vi "Persistent_New_6x8x6.vi"(0 "reference in":refnum<class "G4BaseTemplate_Simple_4x4x4.lvclass">, 1 "Object name":string, 5 "error in (no error)":errorcluster, 6 "CreateMethod(Create or look up existing)":T1(ring), 7 "Persistent/Debugging(Default)":enum16{"Default", "Persistent", "NonPersistent"}(ring)) -> (14 "reference out":refnum<class "G4BaseTemplate_Simple_4x4x4.lvclass">, 15 "NewObjectCreated":bool, 16 "DVRRefOut":refnum<data-value>, 19 "error out":errorcluster)   [LabVIEW 2014]
doc: "..\\..\\..\\..\\Provider_EndevoGOOP400\\Templates\\G4BaseTemplate_Simple_4x4x4\\G4BaseTemplate_Simple_4x4x4.lvclass"
uses:
  <resource>/Framework/Providers/Open_GDS/ClassProviders/Provider_EndevoGOOP400/Templates/G4BaseTemplate_Simple_4x4x4/G4BaseTemplate_Simple_4x4x4.lvclass
  <resource>/Framework/Providers/Open_GDS/ClassProviders/Provider_EndevoGOOP400/Templates/G4BaseTemplate_Simple_4x4x4/protected/ObjectAttributes.ctl
panel:
  in  "DVRRef(Hidden)":refnum<data-value>
  in  "Data":T2 {"Attribute1" format="%.2f"}
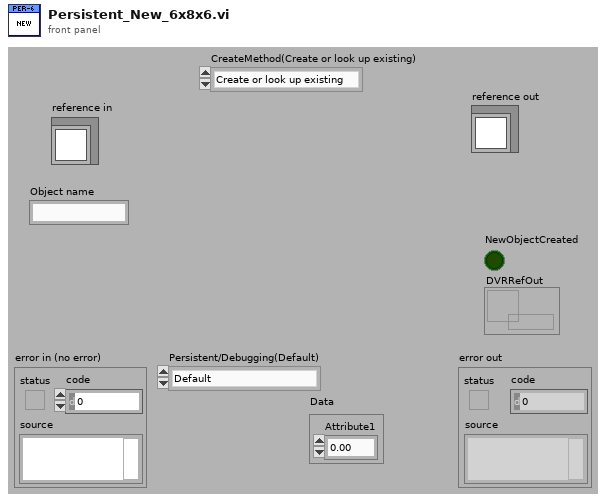
[diagram p1: front panel]
types:
  T1 = enum16{"Create or look up existing", "Look up existing"}
  T2 = typedef "G4BaseTemplate_Simple_4x4x4.lvclass/ObjectAttributes.ctl" = cluster{"Attribute1":dbl}
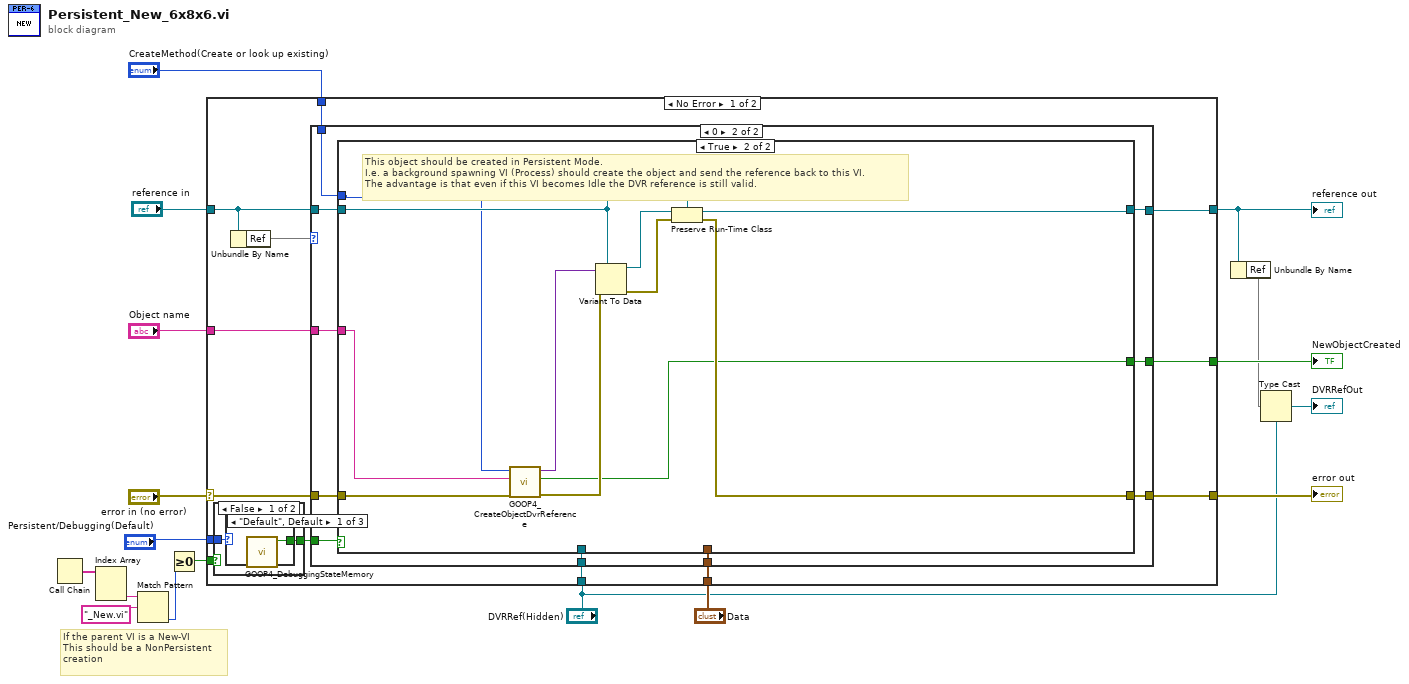
[diagram p0: block diagram]
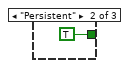
[diagram p2: hidden frame]
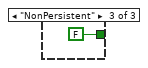
[diagram p3: hidden frame]
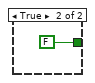
[diagram p4: hidden frame]
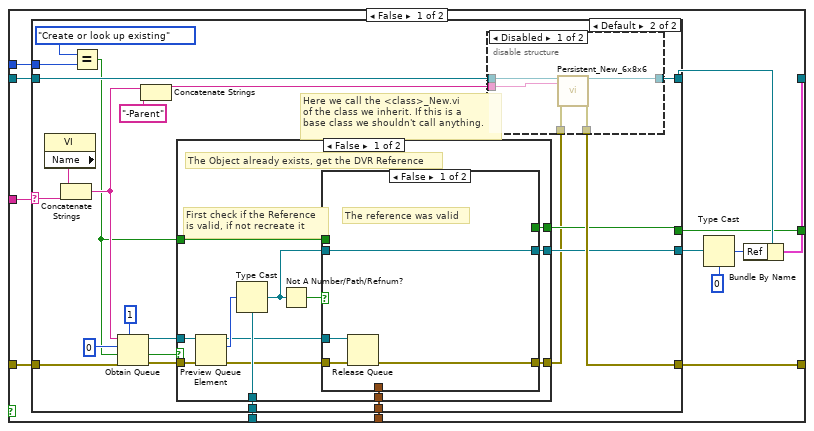
[diagram p6: hidden frame]
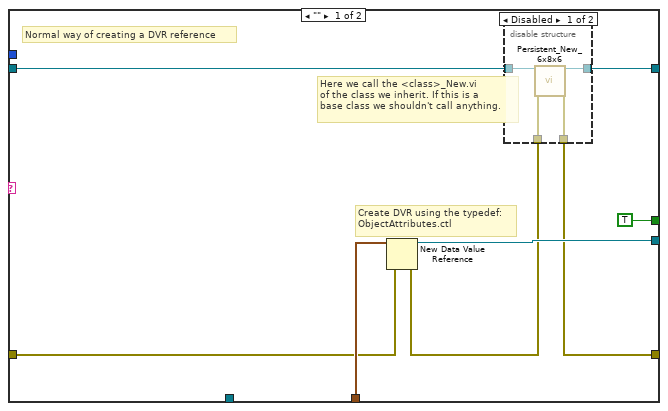
[diagram p7: hidden frame]
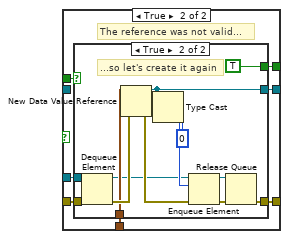
[diagram p9: hidden frame]
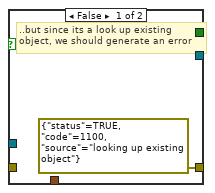
[diagram p10: hidden frame]
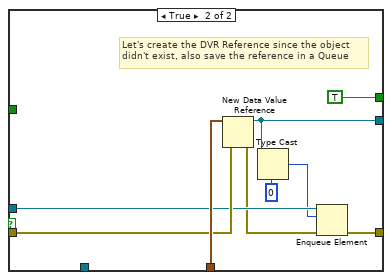
[diagram p11: hidden frame]
diagram:
  # "If the parent VI is a New-VI\nThis should be a NonPersistent\ncreation"
  n1 = Call Chain() -> (call chain=w15:string[])
  n2 = Index Array(array=w15) -> (element #2=w16:string)  [unwired: 2 in, 1 out]
  n3 = Match Pattern(string=w16, regular expression="_New.vi") -> (offset past match=w14:i32)  [unwired: 1 in, 3 out]
  n4 = Greater Or Equal To 0?(x=w14) -> (x >= 0?=w6:bool)
  n5 = case shown="No Error" "error in (no error)" {
    selector: "error in (no error)" -> [w30 w164]
    tunnel: [w27 w164] -> w8
    tunnel: "CreateMethod(Create or look up existing)" -> [w28 _]
    tunnel: "Object name" -> [w29 _]
    tunnel: "Data" -> [w26 _]
    tunnel: "DVRRef(Hidden)" -> [w25 _]
    tunnel: "reference in" -> [w19 w163]
    tunnel: [w24 w163] -> w3
    tunnel: "Persistent/Debugging(Default)" -> [w22 _]
    tunnel: w6 -> [w21 _]
    tunnel: [w20 _] -> w5
    frame No Error {
      n6 = case shown="False" w21 {
        tunnel: w22 -> [w32 _]
        tunnel: [w31 FALSE ("CurrentDebuggingState")] -> w23
        frame False {
          n7 = case shown="\"Default\", Default" w32 {
            tunnel: [w33 TRUE ("CurrentDebuggingState") FALSE ("CurrentDebuggingState")] -> w31
            frame "Default", Default {
              n8 = call <vilib>:"GOOP4_DebuggingStateMemory.vi"() -> ("CurrentDebuggingState"=w33:bool)  [unwired: 10 in, 1 out]
            }
            frame "Persistent" {
            }
            frame "NonPersistent" {
            }
          }
        }
        frame True {
        }
      }
      n9 = Unbundle By Name(w19) -> ("Ref"=w18)
      n10 = case shown="0" w18 {
        tunnel: w30 -> [w38 w48]
        tunnel: w29 -> [_ w47]
        tunnel: w28 -> [_ w46]
        tunnel: [w38 w45] -> w27
        tunnel: w26 -> [_ w44]
        tunnel: w19 -> [w37 w42]
        tunnel: [w37 w43] -> w24
        tunnel: w25 -> [_ w41]
        tunnel: w23 -> [_ w40]
        tunnel: [_ w39] -> w20
        frame Default {
          # "The DVR reference has already been created, from this child class's <Child>_New.vi"
        }
        frame 0 {
          n11 = case shown="True" w40 {
            tunnel: w48 -> [w61 w156]
            tunnel: w47 -> [w60 w152]
            tunnel: w46 -> [w59 w153]
            tunnel: [w58 w157] -> w45
            tunnel: w44 -> [w57 _]
            tunnel: [w56 w158] -> w43
            tunnel: w42 -> [w55 w159]
            tunnel: w41 -> [w53 _]
            tunnel: [w52 w154] -> w39
            frame False {
              n12 = case shown="Default" w60 {
                selector: w60 -> [_ w87]
                tunnel: w61 -> [w68 w96]
                tunnel: [w63 w91] -> w58
                tunnel: w59 -> [_ w95]
                tunnel: w57 -> [w69 w84]
                tunnel: [w67 w83] -> w50
                tunnel: w55 -> [w66 w94]
                tunnel: [w65 w93] -> w54
                tunnel: w53 -> [_ w85]
                tunnel: [TRUE w78] -> w52
                frame "" {
                  # "Create DVR using the typedef:\nObjectAttributes.ctl"
                  # "Here we call the <class>_New.vi\nof the class we inherit. If this is a\nbase class we shouldn't call anything."
                  # "Normal way of creating a DVR reference"
                  n13 = New Data Value Reference(data value=w69, error in=w68) -> (data value reference=w67:refnum<data-value>, error out=w64:errorcluster)
                  n14 = disable-structure shown="Disabled" {
                    disable-tunnel: w66 -> [w73 w75]
                    disable-tunnel: [w72 w75] -> w65
                    disable-tunnel: w64 -> [w71 w74]
                    disable-tunnel: [w70 w74] -> w63
                    frame Disabled {
                      n15 = call <resource>:"Persistent_New_6x8x6.vi"("reference in"=w73, "error in (no error)"=w71) -> ("reference out"=w72:refnum<class "G4BaseTemplate_Simple_4x4x4.lvclass">, "error out"=w70:errorcluster)  [unwired: 14 in, 2 out]
                    }
                    frame Enabled {
                    }
                  }
                }
                frame Default {
                  # "Here we call the <class>_New.vi\nof the class we inherit. If this is a\nbase class we shouldn't call anything."
                  n16 = property class="VI"() -> ("Name"=w88:string)  [unwired: 2 in, 2 out]
                  n17 = Concatenate Strings(w88, w87) -> (w86:string)
                  n18 = Equal?(x=T1."Create or look up existing", y=w95) -> (x = y?=w79:bool)
                  n19 = Obtain Queue(max queue size (-1, unlimited)=1, name (unnamed)=w86, element data type=u32 0 ("DataRef"), create if not found? (T)=w79, error in (no error)=w96) -> (queue out=w82:refnum<queue>, created new?=w80:bool, error out=w81:errorcluster)
                  n20 = Concatenate Strings(w86, "-Parent" ("string")) -> (w89:string)
                  n21 = case shown="False" w80 {
                    tunnel: w81 -> [w109 w143]
                    tunnel: w84 -> [w100 w144]
                    tunnel: w82 -> [w110 w142]
                    tunnel: [w104 w139] -> w77
                    tunnel: [w102 w138] -> w83
                    tunnel: w85 -> [w107 _]
                    tunnel: [w99 TRUE] -> w78
                    tunnel: w79 -> [w98 _]
                    frame False {
                      # "First check if the Reference\nis valid, if not recreate it"
                      # "The Object already exists, get the DVR Reference"
                      n22 = Preview Queue Element(queue=w110, error in (no error)=w109) -> (queue out=w101:refnum<queue>, element=w108:u32, error out=w106:errorcluster)  [unwired: 1 in, 1 out]
                      n23 = Type Cast(type=w107, x=w108) -> (*(type *) &x=w103:refnum<data-value>)
                      n24 = Not A Number/Path/Refnum?(number/path/refnum=w103) -> (NaN/Path/Refnum?=w105:bool)
                      n25 = case shown="False" w105 {
                        tunnel: w106 -> [w112 w120]
                        tunnel: [w111 w117] -> w104
                        tunnel: w103 -> [w114 _]
                        tunnel: [w114 w118] -> w102
                        tunnel: w101 -> [w113 w121]
                        tunnel: w100 -> [_ w119]
                        tunnel: [_ w116] -> w99
                        tunnel: w98 -> [_ w115]
                        frame False {
                          # "The reference was valid"
                          n26 = Release Queue(queue=w113, error in (no error)=w112) -> (error out=w111:errorcluster)  [unwired: 1 in, 2 out]
                        }
                        frame True {
                          # "The reference was not valid..."
                          n27 = case shown="True" w115 {
                            tunnel: w121 -> [_ w135]
                            tunnel: w120 -> [_ w134]
                            tunnel: w119 -> [_ w130]
                            tunnel: [_ w127] -> w118
                            tunnel: [errorcluster {"status"=TRUE, "code"=1100, "source"="looking up existing object"} ("error out") w124] -> w117
                            tunnel: [_ TRUE] -> w116
                            frame False {
                              # "..but since its a look up existing\nobject, we should generate an error"
                            }
                            frame True {
                              # "...so let's create it again"
                              n28 = Dequeue Element(queue=w135, error in (no error)=w134) -> (queue out=w128:refnum<queue>, error out=w131:errorcluster)  [unwired: 1 in, 2 out]
                              n29 = New Data Value Reference(data value=w130, error in=w131) -> (data value reference=w127:refnum<data-value>, error out=w129:errorcluster)
                              n30 = Type Cast(type=u32 0 ("ObjectQueue"), x=w127) -> (*(type *) &x=w132:u32)
                              n31 = Enqueue Element(queue=w128, element=w132, error in (no error)=w129) -> (queue out=w123:refnum<queue>, error out=w125:errorcluster)  [unwired: 1 in, 1 out]
                              n32 = Release Queue(queue=w123, error in (no error)=w125) -> (error out=w124:errorcluster)  [unwired: 1 in, 2 out]
                            }
                          }
                        }
                      }
                    }
                    frame True {
                      # "Let's create the DVR Reference since the object\ndidn't exist, also save the reference in a Queue"
                      n33 = New Data Value Reference(data value=w144, error in=w143) -> (data value reference=w138:refnum<data-value>, error out=w140:errorcluster)
                      n34 = Type Cast(type=u32 0 ("ObjectQueue"), x=w138) -> (*(type *) &x=w137:u32)
                      n35 = Enqueue Element(queue=w142, element=w137, error in (no error)=w140) -> (error out=w139:errorcluster)  [unwired: 1 in, 2 out]
                    }
                  }
                  n36 = disable-structure shown="Disabled" {
                    disable-tunnel: w94 -> [w149 w151]
                    disable-tunnel: [w148 w151] -> w93
                    disable-tunnel: w89 -> [w147 _]
                    disable-tunnel: w77 -> [w146 w150]
                    disable-tunnel: [w145 w150] -> w91
                    frame Disabled {
                      n37 = call <resource>:"Persistent_New_6x8x6.vi"("reference in"=w149, "Object name"=w147, "error in (no error)"=w146) -> ("reference out"=w148:refnum<class "G4BaseTemplate_Simple_4x4x4.lvclass">, "error out"=w145:errorcluster)  [unwired: 13 in, 2 out]
                    }
                    frame Enabled {
                    }
                  }
                }
              }
              n38 = Type Cast(type=u32 0 ("DataRef"), x=w50) -> (*(type *) &x=w49:u32)
              n39 = Bundle By Name(cluster=w54, "Ref"=w49) -> (w56:cluster{})
            }
            frame True {
              # "This object should be created in Persistent Mode.\nI.e. a background spawning VI (Process) should create the object and send the reference back to this VI.\nThe advantage is that even if this VI becomes Idle the DVR reference is still valid."
              n40 = call <vilib>:"GOOP4_CreateObjectDvrReference.vi"("error IO"=w156, "Object name"=w152, "CreateMethod(Create or look up existing)"=w153) -> ("error out"=w155:errorcluster, "created new?"=w154:bool, "ObjectReferenceAsVariant"=w162:variant)  [unwired: 6 in]
              n41 = Variant To Data(error in=w155, type=w159, Variant=w162) -> (data=w161:refnum<class "G4BaseTemplate_Simple_4x4x4.lvclass">, error out=w160:errorcluster)
              n42 = Preserve Run-Time Class(object in=w161, error in=w160, 2:w159) -> (object out=w158:refnum<class "G4BaseTemplate_Simple_4x4x4.lvclass">, error out=w157:errorcluster)
            }
          }
        }
      }
    }
    frame Error {
    }
  }
  "error out" <- w8
  "reference out" <- w3
  "NewObjectCreated" <- w5
  n43 = Unbundle By Name(w3) -> ("Ref"=w4)
  n44 = Type Cast(type="DVRRef(Hidden)", x=w4) -> (*(type *) &x=→"DVRRefOut":refnum<data-value>)
